vi "GetTypeInfo.vi"(8 "Error In":errorcluster, 11 "Variant":variant) -> (0 "Error Out":errorcluster, 1 "HasTypedef":bool, 2 "Name":string, 3 "Type Enum":T1)   [LabVIEW 2016, in "Configit.lvlib"]
doc: "Return information about the datatype stored in Variant.\nType Enum is the type of data\nName is the name of the data\nIf the data is defined by a Type Definition, HasTypedef is true and Typedef contains information about the Type Definition."
uses:
  Configit.lvlib
  <vilib>/Utility/VariantDataType/Type.ctl
  <vilib>/Utility/VariantDataType/VariantType.lvlib
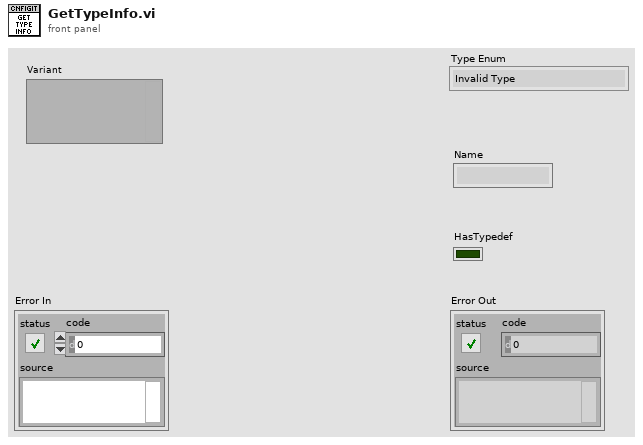
[diagram p1: front panel]
types:
  T1 = typedef "VariantType.lvlib/Type.ctl" = enum8{"Invalid Type", "Void", "I8", "I16", "I32", "I64", "U8", "U16", "U32", "U64", "Single Float", "Double Float", "Extended Float", "Single Complex", "Double Complex", "Extended Complex", "Enum U8", "Enum U16", "Enum U32", "Enum U64", "Single Float With Unit", "Double Float With Unit", "Extended Float With Unit", "Single Complex with Unit", "Double Complex with Unit", "Extended Complex with Unit", "Boolean", "String", "Path", "Picture", "Tag", "Array", "Cluster", "Variant", "LV Variant", "Waveform", "Timestamp", "Digital Waveform", "Digital Data", "ExpressData", "Refnum", "External Data", "VI", "Poly VI", "LabVIEW Class Instance", "Fixed Point"}
  T2 = enum16{"Generic", "Datalog", "ByteStream", "Device", "Occurence", "TCPNetConnection", "OldVisa", "Auto", "LVObj", "Menu", "OldIVI", "Imaq", "Hardware", "DataSocket", "Visa", "IVI", "UDPNetConnection", "Notifier", "Queue", "Irda", "GenClass", "GenClassTag", "DAQmx", "EventReg", "DotNet", "UserEvent", "GenClassDeepCopy", "Callback", "GenClassFlatten", "GenClassTagFlatten", "LVClassInst", "BlueToothNetConnection", "DataValue", "RT FIFO", "TDMS File"}
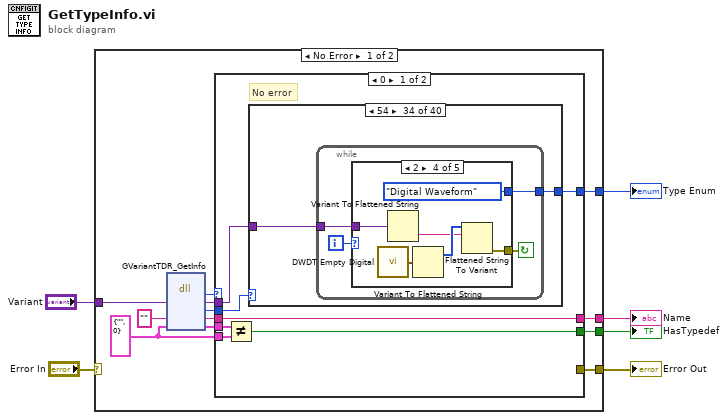
[diagram p0: block diagram]
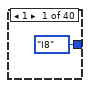
[diagram p2: hidden frame]
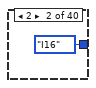
[diagram p3: hidden frame]
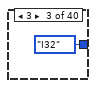
[diagram p4: hidden frame]
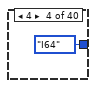
[diagram p5: hidden frame]
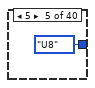
[diagram p6: hidden frame]
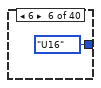
[diagram p7: hidden frame]
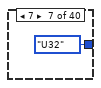
[diagram p8: hidden frame]
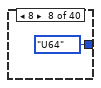
[diagram p9: hidden frame]
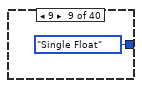
[diagram p10: hidden frame]
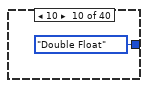
[diagram p11: hidden frame]
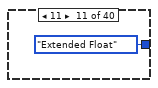
[diagram p12: hidden frame]
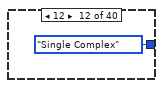
[diagram p13: hidden frame]
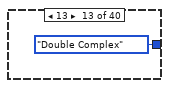
[diagram p14: hidden frame]
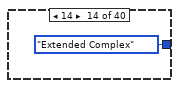
[diagram p15: hidden frame]
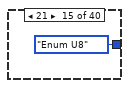
[diagram p16: hidden frame]
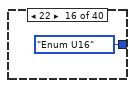
[diagram p17: hidden frame]
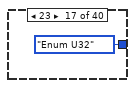
[diagram p18: hidden frame]
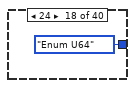
[diagram p19: hidden frame]
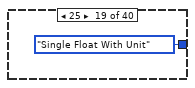
[diagram p20: hidden frame]
diagram:
  n1 = case shown="No Error" "Error In" {
    selector: "Error In" -> [_ w105]
    tunnel: [w18 _] -> w6
    tunnel: [w17 _] -> w5
    tunnel: [w16 _] -> w4
    tunnel: "Variant" -> [w15 _]
    tunnel: [w14 w105] -> w2
    frame No Error {
      w13 = cluster{"Name":string, "Timestamp":u32} {"Name"="", "Timestamp"=0} ("TypedefInfo")
      n2 = dll-call lib="LabVIEW" fn="GVariantTDR_GetInfo"("lvVar"=w15, "name"="", "typeDef"=w13) -> ("return type"=w12:i32, "lvVar"=w7:variant, "typeCode"=w11:i16, "name"=w10:string, "typeDef"=w9:cluster{"Name":string, "Timestamp":u32})  [unwired: 3 in, 3 out]
      n3 = case shown="0" w12 {
        selector: w12 -> [_ w103]
        tunnel: w11 -> [w20 _]
        tunnel: w10 -> [w25 _]
        tunnel: w9 -> [w23 _]
        tunnel: [w21 _] -> w18
        tunnel: [w25 _] -> w17
        tunnel: w13 -> [w24 _]
        tunnel: [w22 _] -> w16
        tunnel: [_ w101] -> w14
        tunnel: w7 -> [w19 _]
        frame 0 {
          # "No error"
          n4 = Not Equal?(x=w23, y=w24) -> (x != y?=w22:bool)
          n5 = case shown="54" w20 {
            tunnel: [Type."I8" ("Type Enum") Type."I16" ("Type Enum") Type."I32" ("Type Enum") Type."I64" ("Type Enum") Type."U8" ("Type Enum") Type."U16" ("Type Enum") Type."U32" ("Type Enum") Type."U64" ("Type Enum") Type."Single Float" ("Type Enum") Type."Double Float" ("Type Enum") Type."Extended Float" ("Type Enum") Type."Single Complex" ("Type Enum") Type."Double Complex" ("Type Enum") Type."Extended Complex" ("Type Enum") Type."Enum U8" ("Type Enum") Type."Enum U16" ("Type Enum") Type."Enum U32" ("Type Enum") Type."Enum U64" ("Type Enum") Type."Single Float With Unit" ("Type Enum") Type."Double Float With Unit" ("Type Enum") Type."Extended Float With Unit" ("Type Enum") Type."Single Complex with Unit" ("Type Enum") Type."Double Complex with Unit" ("Type Enum") Type."Extended Complex with Unit" ("Type Enum") Type."Boolean" ("Type Enum") Type."String" ("Type Enum") Type."Path" ("Type Enum") Type."Picture" ("Type Enum") Type."Tag" ("Type Enum") Type."Array" ("Type Enum") Type."Cluster" ("Type Enum") Type."Variant" ("Type Enum") Type."LV Variant" ("Type Enum") w59 w94 Type."External Data" ("Type Enum") Type."VI" ("Type Enum") Type."Poly VI" ("Type Enum") Type."Fixed Point" ("Type Enum") _] -> w21
            tunnel: w19 -> [_ _ _ _ _ _ _ _ _ _ _ _ _ _ _ _ _ _ _ _ _ _ _ _ _ _ _ _ _ _ _ _ _ w60 w88 _ _ _ _ _]
            frame 1 {
            }
            frame 2 {
            }
            frame 3 {
            }
            frame 4 {
            }
            frame 5 {
            }
            frame 6 {
            }
            frame 7 {
            }
            frame 8 {
            }
            frame 9 {
            }
            frame 10 {
            }
            frame 11 {
            }
            frame 12 {
            }
            frame 13 {
            }
            frame 14 {
            }
            frame 21 {
            }
            frame 22 {
            }
            frame 23 {
            }
            frame 24 {
            }
            frame 25 {
            }
            frame 26 {
            }
            frame 27 {
            }
            frame 28 {
            }
            frame 29 {
            }
            frame 30 {
            }
            frame 33 {
            }
            frame 48 {
            }
            frame 50 {
            }
            frame 51 {
            }
            frame 55 {
            }
            frame 64, 79 {
            }
            frame 80 {
            }
            frame 82 {
            }
            frame 83 {
            }
            frame 84 {
              n6 = while {
                tunnel: [w62] -> w59
                tunnel: w60 -> [w61]
                i -> [w64]
                stop <- w63 continue-if-true
                n7 = case shown="2" w64 {
                  tunnel: w61 -> [_ w67 w72 w79 w85]
                  tunnel: [_ w66 w70 w76 w82] -> w63
                  tunnel: [Type."Invalid Type" ("Type Enum") Type."Timestamp" ("Type Enum") Type."Waveform" ("Type Enum") Type."Digital Waveform" ("Type Enum") Type."Digital Data" ("Type Enum")] -> w62
                  frame Default {
                  }
                  frame 0 {
                    n8 = Variant To Data(type=timestamp(0 s since 1904-01-01), Variant=w67) -> (error out=w66:errorcluster)  [unwired: 1 in, 1 out]
                  }
                  frame 1 {
                    n9 = Variant To Data(type=waveform(dbl) {"t0"=timestamp(0 s since 1904-01-01), "dt"=0.0, "Y"=[]} ("Waveform 2"), Variant=w72) -> (error out=w70:errorcluster)  [unwired: 1 in, 1 out]
                  }
                  frame 2 {
                    n10 = call <vilib>:"DWDT Empty Digital.vi"() -> ("digital waveform out"=w74:digitalwaveform)  [unwired: 5 in]
                    n11 = Variant To Flattened String(Variant=w79) -> (data string=w77:string)  [unwired: 1 out]
                    n12 = Variant To Flattened String(Variant=w74) -> (1:w78:i16[])  [unwired: 1 out]
                    n13 = Flattened String To Variant(6:w77, 7:w78) -> (0:w76:errorcluster)  [unwired: 1 in, 1 out]
                  }
                  frame 3 {
                    n14 = call <vilib>:"DTbl Empty Digital.vi"() -> ("digital data"=w80:digitaldata)  [unwired: 5 in]
                    n15 = Variant To Flattened String(Variant=w85) -> (data string=w83:string)  [unwired: 1 out]
                    n16 = Variant To Flattened String(Variant=w80) -> (1:w84:i16[])  [unwired: 1 out]
                    n17 = Flattened String To Variant(6:w83, 7:w84) -> (0:w82:errorcluster)  [unwired: 1 in, 1 out]
                  }
                }
              }
            }
            frame 112 {
              n18 = dll-call lib="LabVIEW" fn="GVariantTDR_GetRefnumInfo"("lvVar"=w88, "regNumKind"=i16 0 ("refNumKind"), "subKind"=0, "innerType"=variant ("Variant"), "info"="") -> ("regNumKind"=w92:i16)  [unwired: 4 in, 6 out]
              n19 = Type Cast(type=T2."Generic" ("Refnum Kind"), x=w92) -> (*(type *) &x=w87:T2)
              n20 = case shown="\"LVClassInst\"" w87 {
                tunnel: [Type."Refnum" ("Type Enum 2") Type."LabVIEW Class Instance" ("Type Enum 2")] -> w94
                frame Default {
                }
                frame "LVClassInst" {
                }
              }
            }
            frame 132 {
            }
            frame 240 {
            }
            frame 242 {
            }
            frame 95 {
            }
            frame Default {
            }
          }
        }
        frame Default {
          # "Error"
          n21 = Bundle("status"=TRUE, w103, "") -> (w101:cluster{"status":bool, i32, string})  [unwired: 1 in]
        }
      }
    }
    frame Error {
    }
  }
  "Type Enum" <- w6
  "Name" <- w5
  "HasTypedef" <- w4
  "Error Out" <- w2
